vi "SimpleCurveAdded Event Callback.vi"(4 "User Parameter":T2, 5 "Event Data":T3, 6 "Control Ref":refnum<k24>, 7 "Event Common Data":T4) -> ()   [LabVIEW 2025]
uses:
  C:/Users/stef/code/palmsenssdk/labview/PalmSens/Libraries/PalmSens.Core.Simplified.LabVIEW.dll
  Libraries/PalmSens.Core.Simplified.LabVIEW.dll
  ActiveCurve.ctl
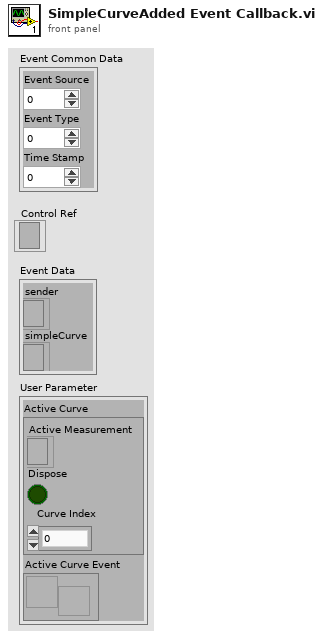
[diagram p1: front panel]
types:
  T1 = typedef "ActiveCurve.ctl" = cluster{"Active Measurement":refnum<k24>, "Dispose":bool, "Curve Index":i32}
  T2 = cluster{"Active Curve":T1, "Active Curve Event":refnum<user-event>}
  T3 = cluster{"sender":refnum<k24>, "simpleCurve":refnum<k24>}
  T4 = cluster{"Event Source":i32, "Event Type":u32, "Time Stamp":u32}
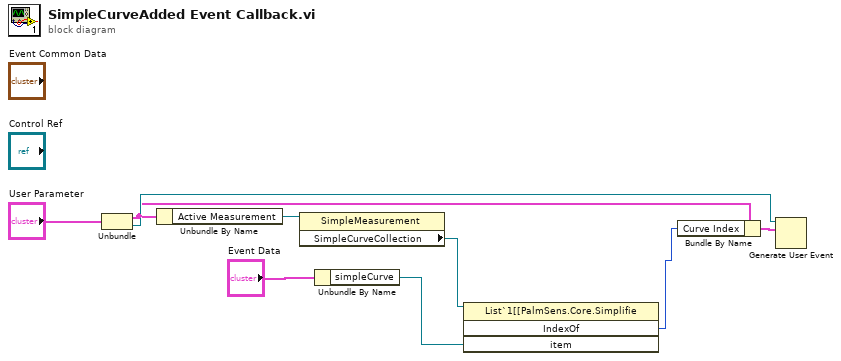
[diagram p0: block diagram]
diagram:
  n1 = Unbundle("User Parameter") -> ("Active Curve"=w5:T1, "Active Curve Event"=w7:refnum<user-event>)
  n2 = Unbundle By Name(w5) -> ("Active Measurement"=w4:refnum<k24>)
  n3 = property class="SimpleMeasurement"(reference=w4) -> ("SimpleCurveCollection"=w3:refnum<k24>)  [unwired: 1 in, 2 out]
  n4 = Unbundle By Name("Event Data") -> ("simpleCurve"=w2:refnum<k24>)
  n5 = invoke class="List`1[[PalmSens.Core.Simplifie" method="IndexOf"(reference=w3, "item"=w2) -> ("IndexOf"=w1:i32)  [unwired: 2 in, 3 out]
  n6 = Bundle By Name(cluster=w5, "Curve Index"=w1) -> (w6:T1)
  n7 = Generate User Event(user event=w7, event data cluster=w6) -> ()  [unwired: 2 in, 2 out]
